vi "database_connection_nowrite_EVO.vi"(5 "ODBC data source name":string="amrc_monitoring", 6 "error in (no error)":errorcluster, 7 "G1?":u32, 8 "current time":timestamp, 9 "data 2":dbl[](array[numeric]), 10 "Machine Data":T1={"Zload"="", "Yload"="", "Xload"="", "path_position"="", "Fovr"="", "SspeedOvr"="", "Program Name"="", "Program status"="", "Block of code being executed"="", "Line of code"="", "Machine availability"="", "Emergency status"="", "Controller mode"="", "Tool_id"="UNAVAILABLE"}, 11 "Machine type":string) -> (3 "error out":errorcluster)   [LabVIEW 2017]
uses:
  <vilib>/regexp/Match Regular Expression.xnode
panel:
  out "data 3":dbl[](array[numeric])
  out "path_position":string
  out "x = y?":bool
  out "submatch 1":string
  out "after match 3":string
  out "empty? 2":bool
  out "after match 2":string
  out "resulting string 4":string
  out "Xload":string
  out "concatenated string 6":string
  out "resulting string 3":string
  out "concatenated string 2":string
  out "resulting string 2":string
  out "ODBC data source name 2":string="amrc_monitoring"
  out "resulting string":string
  out "size(s)":i32
  out "concatenated string 5":string
  out "concatenated string 3":string
  out "concatenated string":string
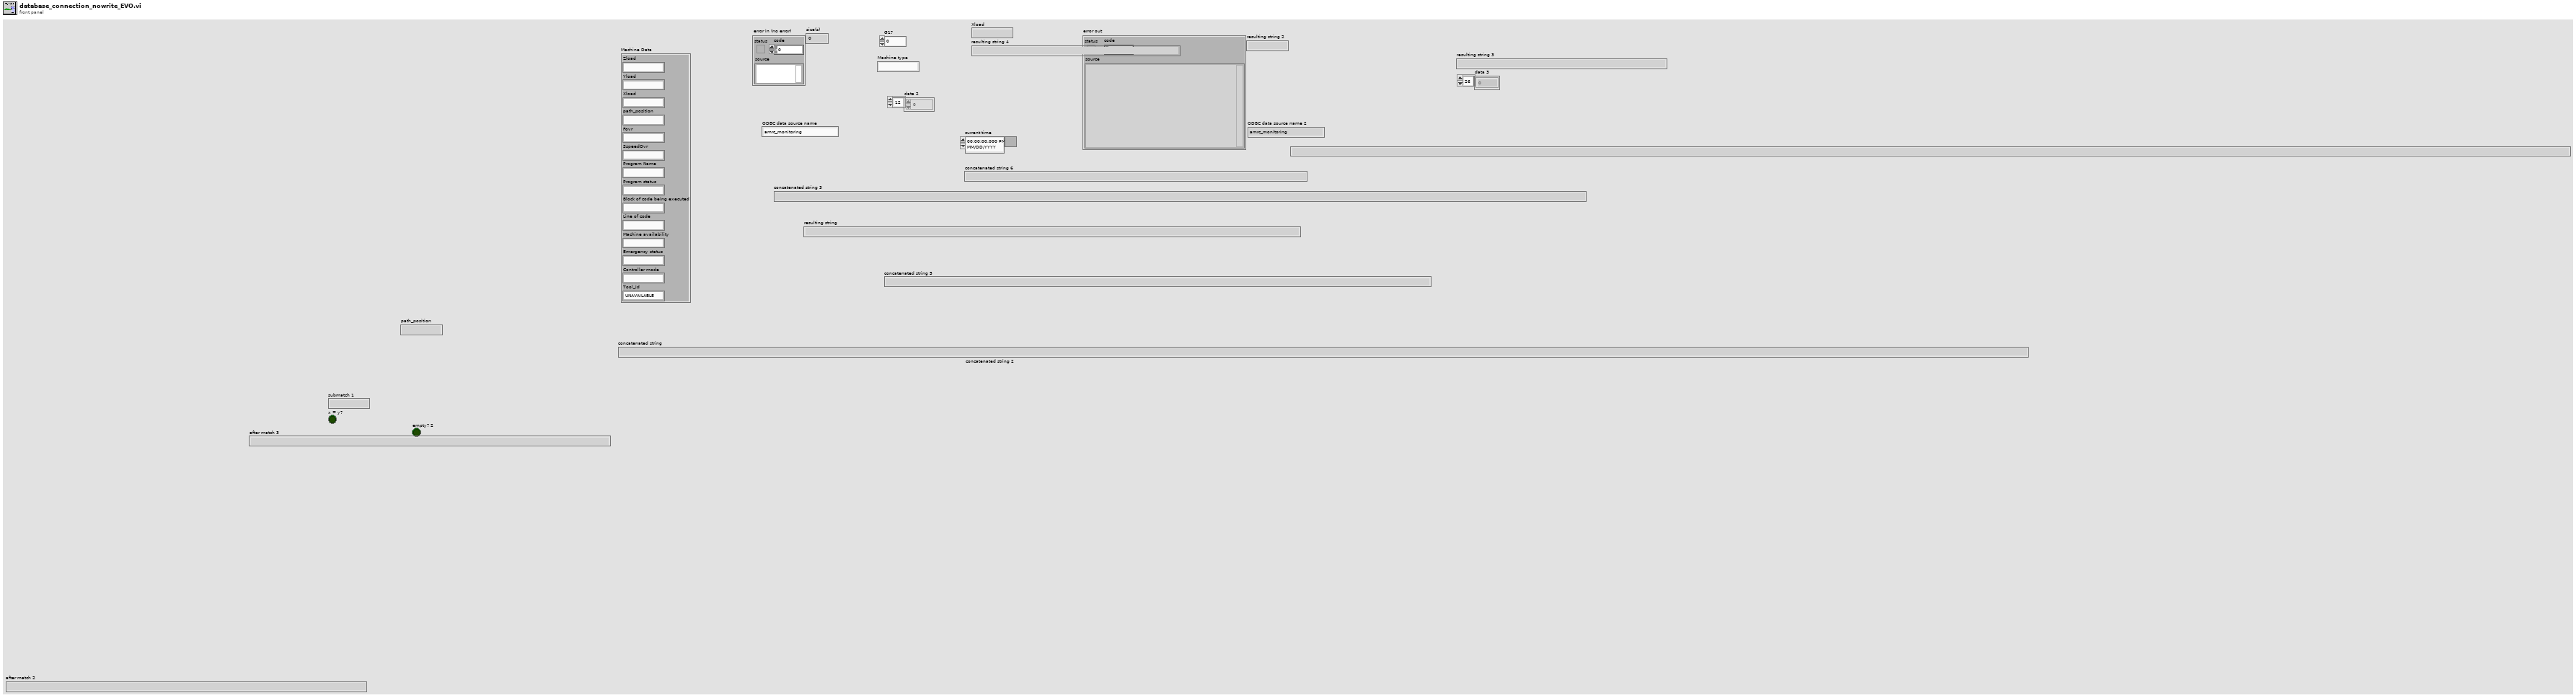
[diagram p1: front panel]
types:
  T1 = cluster{"Zload":string, "Yload":string, "Xload":string, "path_position":string, "Fovr":string, "SspeedOvr":string, "Program Name":string, "Program status":string, "Block of code being executed":string, "Line of code":string, "Machine availability":string, "Emergency status":string, "Controller mode":string, "Tool_id":string}
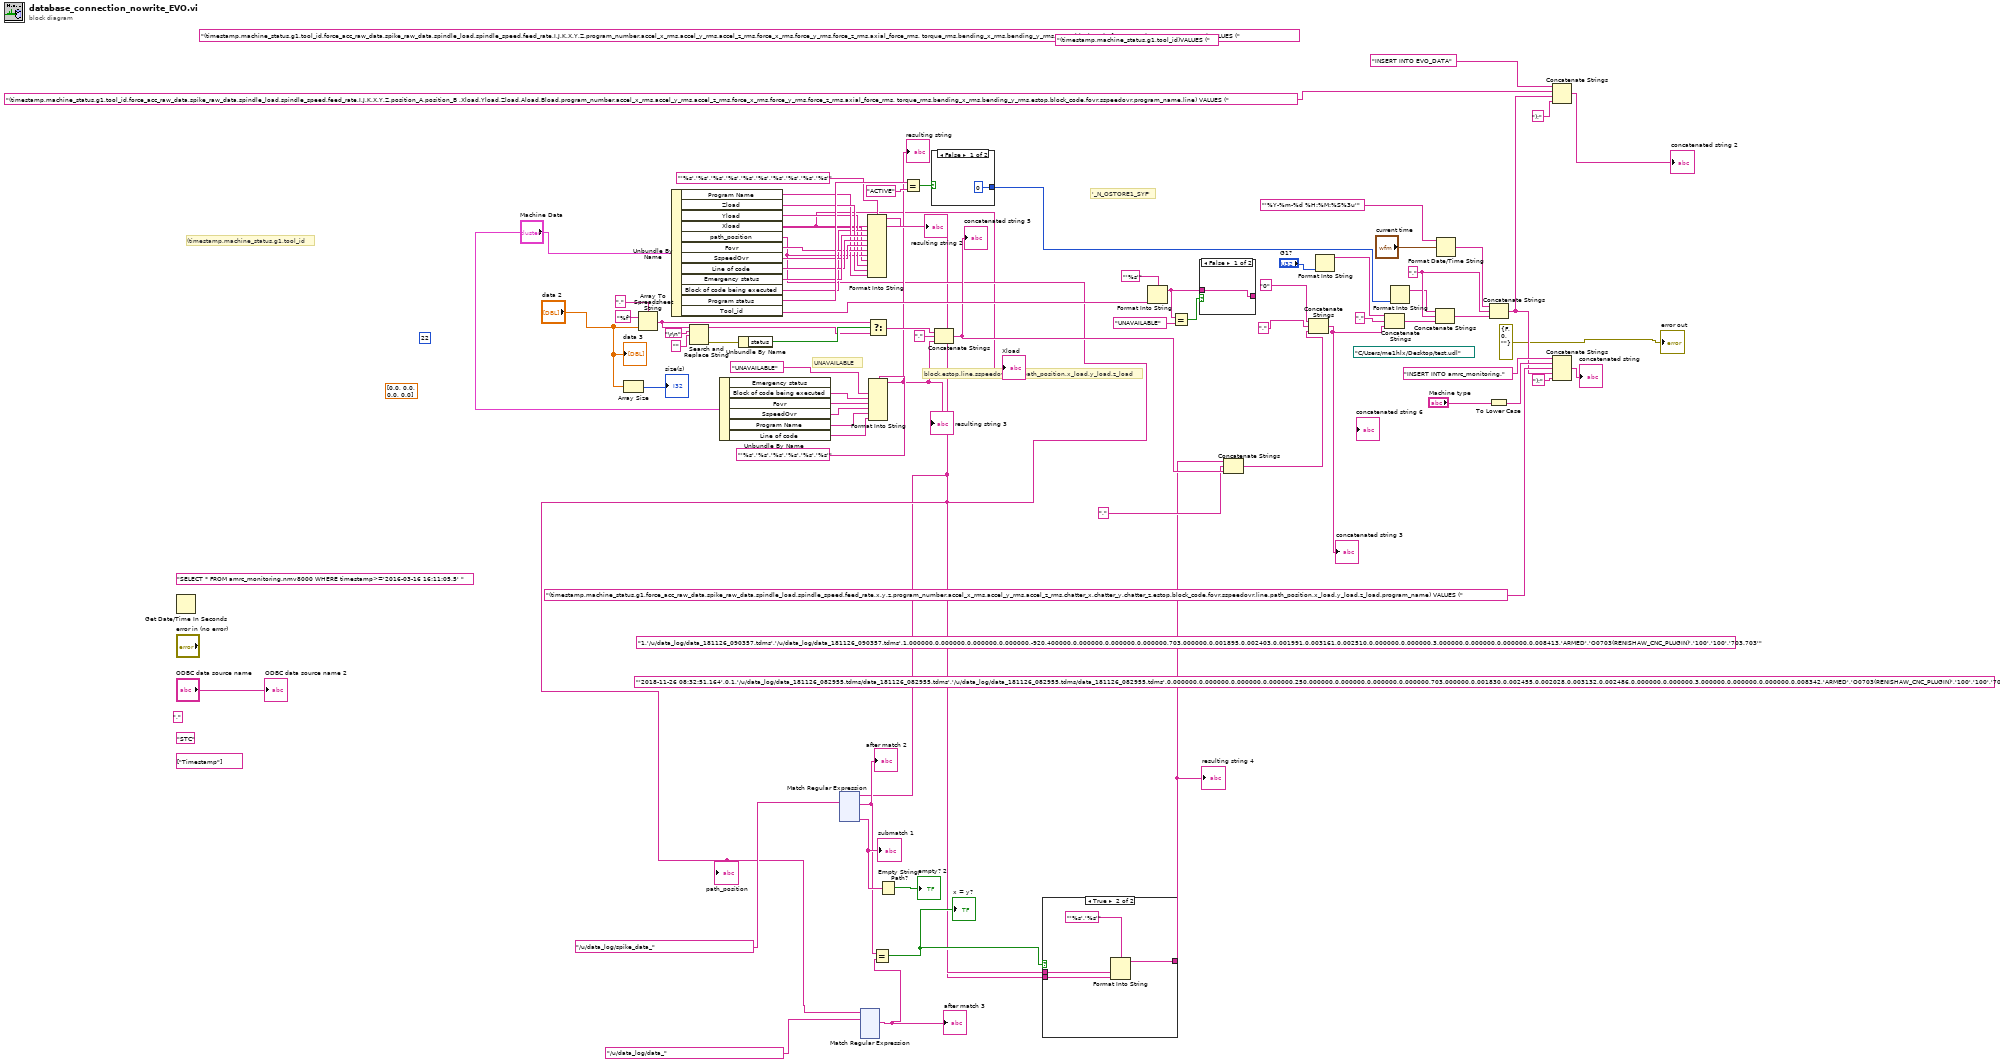
[diagram p0: block diagram]
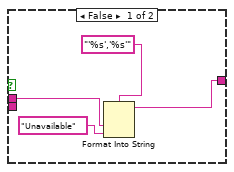
[diagram p2: hidden frame]
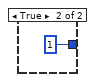
[diagram p4: hidden frame]
diagram:
  (unwired) "(timestamp,machine_status,g1,tool_id,force_acc_raw_data,spike_raw_data,spindle_load,spindle_speed,feed_rate,I,J,K,X,Y,Z,program_number,accel_x_rms,accel_y_rms,accel_z_rms,force_x_rms,force_y_rms,force_z_rms,axial_force_rms, torque_rms,bending_x_rms,bending_y_rms,estop,block_code,fovr,sspeedovr,program_name) VALUES (" ("string")
  (unwired) "(timestamp,machine_status,g1,tool_id)VALUES (" ("string")
  (unwired) dbl[] [0.0, 0.0, 0.0, 0.0]
  (unwired) "1,'/u/data_log/data_181126_090357.tdms','/u/data_log/data_181126_090357.tdms',1.000000,0.000000,0.000000,0.000000,-920.400000,0.000000,0.000000,0.000000,703.000000,0.001895,0.002403,0.001991,0.003161,0.002510,0.000000,0.000000,3.000000,0.000000,0.000000,0.008413,'ARMED','O0703(RENISHAW_CNC_PLUGIN)','100','100','703.703'" ("concatenated string 4")
  (unwired) "'2018-11-26 08:32:51.164',0,1,'/u/data_log/data_181126_082955.tdms/data_181126_082955.tdms','/u/data_log/data_181126_082955.tdms/data_181126_082955.tdms',0.000000,0.000000,0.000000,0.000000,250.000000,0.000000,0.000000,0.000000,703.000000,0.001830,0.002455,0.002028,0.003132,0.002486,0.000000,0.000000,3.000000,0.000000,0.000000,0.008342,'ARMED','O0703(RENISHAW_CNC_PLUGIN)','100','100','703.703'" ("concatenated string 2")
  (unwired) 22
  (unwired) "," ("string")
  (unwired) string[] ["Timestamp"]
  (unwired) "STC"
  (unwired) path "C:/Users/me1hlx/Desktop/test.udl" ("connection information")
  w39 = "," ("string")
  (unwired) "SELECT * FROM amrc_monitoring.nmv8000 WHERE timestamp>='2016-03-16 16:11:05.5' " ("SQL query")
  # "(timestamp,machine_status,g1,tool_id"
  # "'_N_OSTORE1_SYF'"
  # "UNAVAILABLE"
  # "block,estop,line,sspeedovr,fovr,path_position,x_load,y_load,z_load"
  n1 = Get Date/Time In Seconds() -> ()  [unwired: 1 out]
  n2 = Array Size(array="data 2") -> (size(s)=→"size(s)":i32)
  n3 = Array To Spreadsheet String(delimiter (Tab)=",", array="data 2", 3:"%f" ("format string")) -> (spreadsheet string=w64:string)
  n4 = Unbundle By Name("Machine Data") -> ("Program Name"=w51:string, "Zload"=w55:string, "Yload"=w25:string, "Xload"=w4:string, "path_position"=w5:string, "Fovr"=w56:string, "SspeedOvr"=w57:string, "Line of code"=w58:string, "Emergency status"=w59:string, "Block of code being executed"=w49:string, "Program status"=w77:string, "Tool_id"=w43:string)
  "Xload" <- w4
  "path_position" <- w5
  n5 = Search and Replace String(input string=w64, search string="\r\n", replace string="" ("replace string (\"\")")) -> (result string=w65:string, error out=w67:errorcluster)  [unwired: 5 in, 2 out]
  n6 = Unbundle By Name("Machine Data") -> ("Block of code being executed"=w32:string, "Fovr"=w31:string, "SspeedOvr"=w30:string, "Program Name"=w29:string, "Line of code"=w2:string)  [unwired: 1 out]
  n7 = Unbundle By Name(w67) -> ("status"=w66:bool)
  n8 = xnode "Match Regular Expression"("input string"=w4, "regular expression"="/u/data_log/spike_data_") -> ("after match"=w8:string, "submatch 1"=w9:string)  [unwired: 4 in, 4 out]
  "after match 2" <- w8
  "submatch 1" <- w9
  n9 = xnode "Match Regular Expression"("input string"=w5, "regular expression"="/u/data_log/data_") -> ("after match"=w7:string)  [unwired: 4 in, 5 out]
  "after match 3" <- w7
  n10 = Format Into String(format string="'%s','%s','%s','%s','%s','%s','%s','%s','%s','%s'", w49, w59, w58, w57, w56, w5, w4, w25, w55, w51) -> (resulting string=→"resulting string 2":string)  [unwired: 2 in, 1 out]
  n11 = Select(t=w64, s=w66, f=w65) -> (s? t:f=w52:string)
  n12 = Format Into String(format string="'%s','%s','%s','%s','%s','%s'", "UNAVAILABLE" ("format string"), w32, w31, w30, w29, w2) -> (resulting string=w24:string)  [unwired: 2 in, 1 out]
  "resulting string" <- w24
  "resulting string 3" <- w24
  n13 = Equal?(x=w8, y=w7) -> (x = y?=w6:bool)
  "x = y?" <- w6
  n14 = Empty String/Path?(string/path=w9) -> (empty?=→"empty? 2":bool)
  n15 = Equal?(x=w77, y="ACTIVE") -> (x = y?=w75:bool)
  n16 = case shown="False" w75 {
    tunnel: [0 1] -> w20
    frame False {
    }
    frame True {
    }
  }
  n17 = Concatenate Strings(w52, "," ("string"), w24) -> (w16:string)
  "concatenated string 5" <- w16
  n18 = case shown="True" w6 {
    tunnel: w5 -> [w84 w86]
    tunnel: w4 -> [_ w89]
    tunnel: [w83 w87] -> w3
    frame False {
      n19 = Format Into String(format string="'%s','%s'", w84, "Unavailable" ("Tool_id")) -> (resulting string=w83:string)  [unwired: 2 in, 1 out]
    }
    frame True {
      n20 = Format Into String(format string="'%s','%s'", w86, w89) -> (resulting string=w87:string)  [unwired: 2 in, 1 out]
    }
  }
  "resulting string 4" <- w3
  n21 = Format Into String(format string="'%s'", w43) -> (resulting string=w42:string)  [unwired: 2 in, 1 out]
  n22 = Equal?(x=w42, y="UNAVAILABLE") -> (x = y?=w74:bool)
  n23 = case shown="False" w74 {
    tunnel: w42 -> [w90 w91]
    tunnel: [w90 w91] -> _
    frame False {
    }
    frame True {
    }
  }
  n24 = Concatenate Strings(w3, "," ("string"), w16) -> (w14:string)
  n25 = Concatenate Strings("0", "," ("string"), w14) -> (w21:string)
  "concatenated string 3" <- w21
  n26 = Format Into String("G1?") -> (resulting string=w37:string)  [unwired: 3 in, 1 out]
  n27 = Concatenate Strings(w37, "," ("string"), w21) -> (w23:string)
  n28 = Format Into String(w20) -> (resulting string=w38:string)  [unwired: 3 in, 1 out]
  n29 = Concatenate Strings(w38, w39, w23) -> (w70:string)
  n30 = Format Date/Time String(time format string (%c)="'%Y-%m-%d %H:%M:%S%3u'", seconds (now)="current time") -> (date/time string=w40:string)  [unwired: 1 in]
  n31 = To Lower Case(string="Machine type") -> (all lower case string=w61:string)
  n32 = Concatenate Strings(w40, w39, w70) -> (w22:string)
  n33 = Concatenate Strings("INSERT INTO EVO_DATA" ("string"), "(timestamp,machine_status,g1,tool_id,force_acc_raw_data,spike_raw_data,spindle_load,spindle_speed,feed_rate,I,J,K,X,Y,Z,position_A,position_B ,Xload,Yload,Zload,Aload,Bload,program_number,accel_x_rms,accel_y_rms,accel_z_rms,force_x_rms,force_y_rms,force_z_rms,axial_force_rms, torque_rms,bending_x_rms,bending_y_rms,estop,block_code,fovr,sspeedovr,program_name,line) VALUES (" ("string"), w22, ");" ("string")) -> (→"concatenated string 2":string)
  n34 = Concatenate Strings("INSERT INTO amrc_monitoring." ("string"), w61, "(timestamp,machine_status,g1,force_acc_raw_data,spike_raw_data,spindle_load,spindle_speed,feed_rate,x,y,z,program_number,accel_x_rms,accel_y_rms,accel_z_rms,chatter_x,chatter_y,chatter_z,estop,block_code,fovr,sspeedovr,line,path_position,x_load,y_load,z_load,program_name) VALUES (" ("string"), w22, ");" ("string")) -> (→"concatenated string":string)
  "error out" <- errorcluster {"status"=FALSE, "code"=0, "source"=""} ("error in (no error)")
  "ODBC data source name 2" <- "ODBC data source name"
  "data 3" <- "data 2"
